vi "HumanDriveAxesProcessing.vi"(8 "Right X":dbl, 9 "Right Y":dbl, 10 "Left X":dbl, 11 "Left Y":dbl) -> (0 "Right X":dbl, 1 "Right Y":dbl, 2 "Left X":dbl, 3 "Left Y":dbl)   [LabVIEW 2023]
uses:
  <vilib>/Rock Robotics/WPI/ThirdParty/JAS_Junk/TrajLib/Trajectory_Library.lvlib
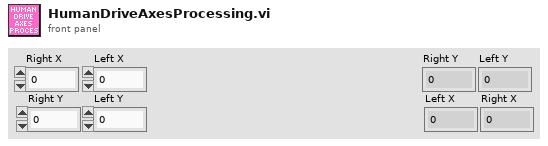
[diagram p1: front panel]
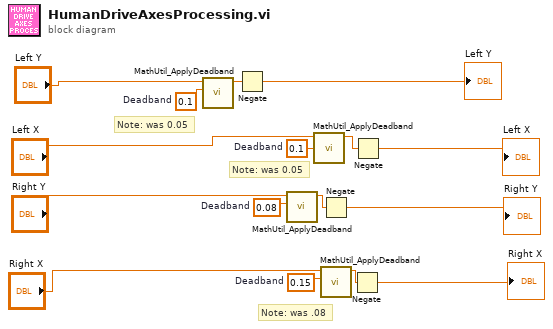
[diagram p0: block diagram]
diagram:
  w9 = 0.15  # Deadband
  w10 = 0.1  # Deadband
  w13 = 0.08  # Deadband
  w16 = 0.1  # Deadband
  # "Note: was .08"
  # "Note: was 0.05"
  # "Note: was 0.05"
  n1 = call <vilib>:"MathUtil_ApplyDeadband.vi"("Deadband"=w16, "Value"="Left Y") -> ("Result"=w15:dbl)  [unwired: 9 in]
  n2 = Negate(x=w15) -> (-x=→"Left Y":dbl)
  n3 = call <vilib>:"MathUtil_ApplyDeadband.vi"("Deadband"=w13, "Value"="Right Y") -> ("Result"=w12:dbl)  [unwired: 9 in]
  n4 = call <vilib>:"MathUtil_ApplyDeadband.vi"("Deadband"=w10, "Value"="Left X") -> ("Result"=w7:dbl)  [unwired: 9 in]
  n5 = Negate(x=w12) -> (-x=→"Right Y":dbl)
  n6 = call <vilib>:"MathUtil_ApplyDeadband.vi"("Deadband"=w9, "Value"="Right X") -> ("Result"=w8:dbl)  [unwired: 9 in]
  n7 = Negate(x=w8) -> (-x=→"Right X":dbl)
  n8 = Negate(x=w7) -> (-x=→"Left X":dbl)
